vi "Jtrans_quart.vi"(1 "eta":dbl[](array[numeric])) -> (0 "J trans":T1)   [LabVIEW 2014]
uses:
  <vilib>/Analysis/Matrix/Datatypes/RealMatrix.ctl
  <vilib>/Analysis/7linalg.llb/Real Transpose Matrix.vi
  TransformationMatrixQuaternions.vi
  RotationMatrixQuaternions.vi
  <vilib>/imath/engines/lvmath2/RunTimeEngine/RowToken/NIMS_RowToken_M_M.vi
  <instcachedir>/0/NIMS_RowToken_M_M_4C96C156B57B4BCFA08E125188784392.lvgen/NIMS_RowToken_M_M_4C96C156B57B4BCFA08E125188784392_004.vi
  <vilib>/imath/engines/lvmath2/RunTimeEngine/MatrixToken/NIMS_MatrixToken_M_M.vi
  <instcachedir>/0/NIMS_MatrixToken_M_M_F8DD6808CBBD42C5992E1D2201A8964A.lvgen/NIMS_MatrixToken_M_M_F8DD6808CBBD42C5992E1D2201A8964A_004.vi
  <vilib>/imath/engines/lvmath2/RunTimeEngine/ErrorHandling/NIMS_Create Error From Enums.vi
  <vilib>/imath/engines/lvmath2/RunTimeEngine/NodeEndStatement/NIMS_NodeEndStatement_Output.vi
  <instcachedir>/0/NIMS_NodeEndStatement_Output_53EC0D466D134D7ABD903AC30B43404B.lvgen/NIMS_NodeEndStatement_Output_53EC0D466D134D7ABD903AC30B43404B_002.vi
  <vilib>/imath/engines/lvmath2/RunTimeEngine/ErrorHandling/NIMS_Finalize Error.vi
  <vilib>/Analysis/NI_AALPro.lvlib
  <vilib>/Analysis/Matrix/NI_Matrix.lvlib
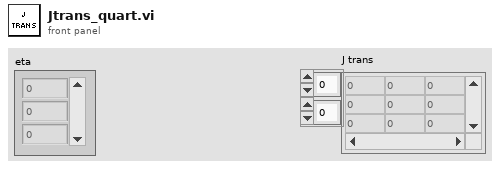
[diagram p1: front panel]
types:
  T1 = typedef "NI_Matrix.lvlib/RealMatrix.ctl" = dbl[][]
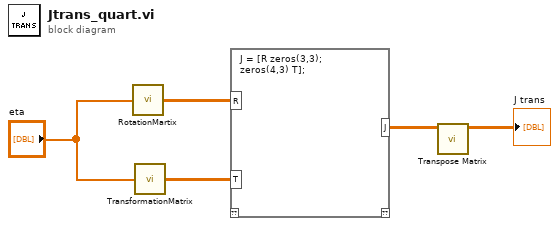
[diagram p0: block diagram]
diagram:
  n1 = call-poly "RotationMartix.vi"("Eta_q"="eta") -> ("R"=w3:dbl[][])
  n2 = call-poly "TransformationMatrix.vi"("Eta_q"="eta") -> ("T_q"=w4:dbl[][])
  n3 = mathscript code="J = [R zeros(3,3);\nzeros(4,3) T];"("R"=w3, "T"=w4) -> ("J"=w2:dbl[][])  [unwired: 1 in, 1 out]
  n4 = call-poly <vilib>:"Transpose Matrix.vi"("Input Matrix"=w2) -> ("Matrix Transpose"=→"J trans":T1)  [unwired: 9 in, 1 out]
